vi "CheckResponse.vi"(5 "+veResponseCode":u8=160 format="%x", 7 "STP CMD":T2=130 items=["TSW_VERSION(130)"=130, "WAIT_EVENT(132)"=132, "SEQUENCER(133)"=133, "TSW_RESET(150)"=150, "CONFIG_ECU(151)"=151, "TEST_CORE (152)"=152, "TEST_WATCHDOG (153)"=153, "TEST_MONITORING (154)"=154, "READ_MEMORY (162)"=162, "WRITE_ERASE_MEMORY (164)"=164, "COMM_EXTERNAL (190)"=190, "COMM_INTERNAL (195)"=195, "GET_ANALOG_INPUT (210)"=210, "GET_DIGITAL_INPUT (211)"=211, "GET_FREQUENCY_INPUT (212)"=212, "TEST_INPUT_STRUCTURE (214)"=214, "GENERATE_OUTPUT_SIGNAL (220)"=220, "GENERATE_SYNCHRONIZED_OUTPUT_SIGNALS (221)"=221, "eDCU_Specific (250)"=250], 9 "STP Loop Data In":T1, 10 "Rx CAN frame":T4 {"payload" format="%x"; "timestamp" format="%<%.7X\n%x>T"; "type" items=["CAN Data"=0, "CAN Remote"=1, "CAN Bus Error"=2, "CAN 2.0 Data"=8, "CAN FD Data"=16, "CAN FD+BRS Data"=24, "J1939 Data"=192, "Delay"=224, "Log Trigger"=225, "Start Trigger"=226]; "identifier" format="%x"}, 11 "RxID":u32=2043 format="%x") -> (1 "STP Loop Data Out":T1, 2 "Valid Response?":bool, 3 "STP_NextState":T3=enum."Check Ack")   [LabVIEW 2023, in "HardwareAbstractionLayer_LVOOP.lvlib" / "CAN Application Protocols Lib.lvlib" / "STP Protocol.lvclass"]
uses:
  STP Protocol.lvclass
  <vilib>/xnet/xnet.llb/XNET Frame CAN.ctl
  <vilib>/xnet/xnet.llb/XNET Frame Type CAN.ctl
  Ctrls/STP States.ctl
  Ctrls/STP CMD.ctl
  Ctrls/STP Loop Data.ctl
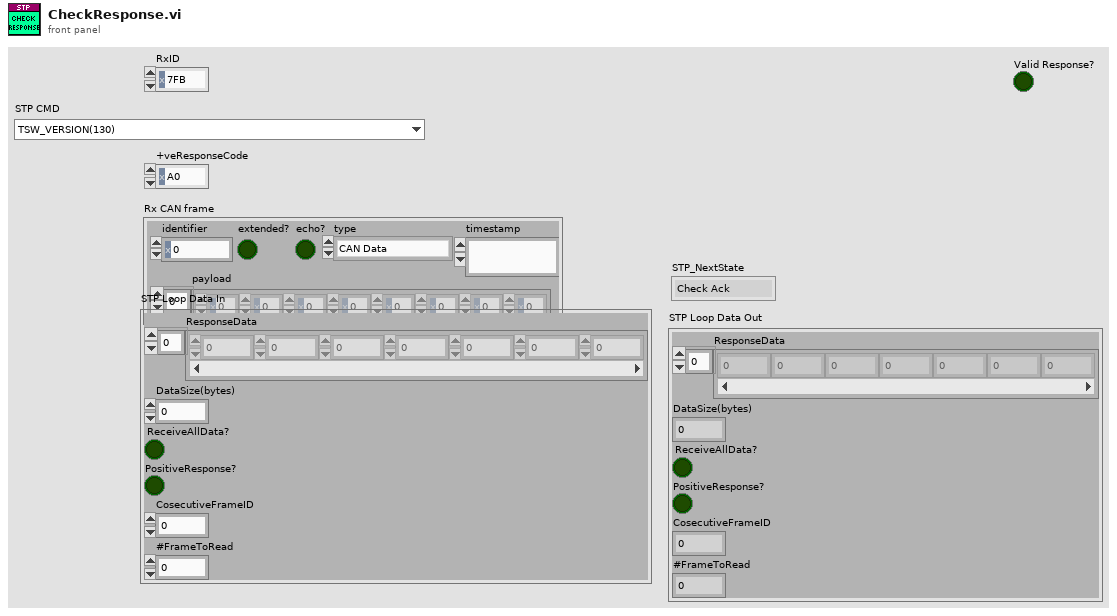
[diagram p1: front panel]
types:
  T1 = typedef "HardwareAbstractionLayer_LVOOP.lvlib/CAN Application Protocols Lib.lvlib/STP Protocol.lvclass/STP Loop Data.ctl" = cluster{"ResponseData":u8[], "DataSize(bytes)":u16, "ReceiveAllData?":bool, "PositiveResponse?":bool, "CosecutiveFrameID":fxp<+,4,4>, "#FrameToRead":i32}
  T2 = typedef "HardwareAbstractionLayer_LVOOP.lvlib/CAN Application Protocols Lib.lvlib/STP Protocol.lvclass/STP CMD.ctl" = u8
  T3 = typedef "HardwareAbstractionLayer_LVOOP.lvlib/CAN Application Protocols Lib.lvlib/STP Protocol.lvclass/STP States.ctl" = enum16{"Init", "Send Request", "Check Ack", "Send TP Frames", "Send Flow Control Frame", "Check Response", "Read TP Data", "Return Data", "Return Positive Response", "Return Error Response", "Exit"}
  T4 = typedef "XNET Frame CAN.ctl" = cluster{"timestamp":timestamp, "payload":u8[], "identifier":u32, "type":T5, "extended?":bool, "echo?":bool}
  T5 = typedef "XNET Frame Type CAN.ctl" = u8
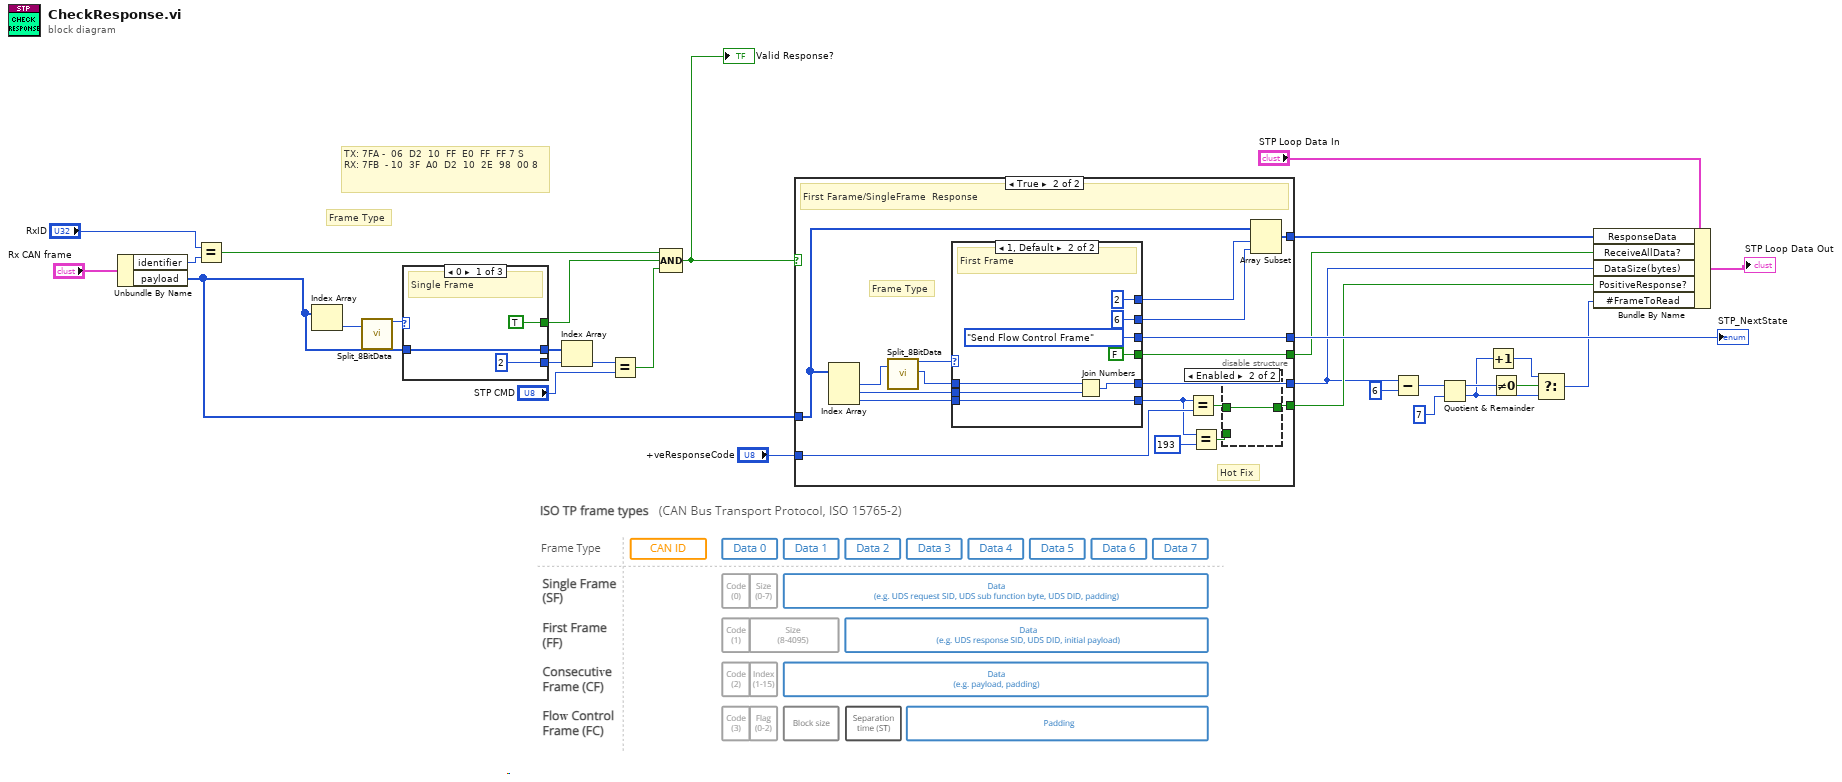
[diagram p0: block diagram]
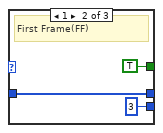
[diagram p2: hidden frame]
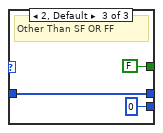
[diagram p3: hidden frame]
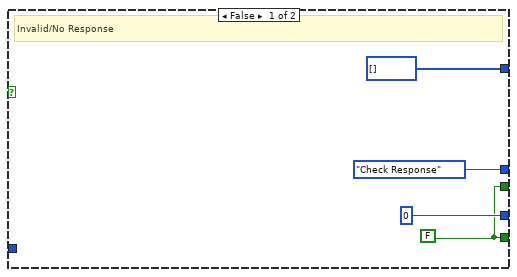
[diagram p4: hidden frame]
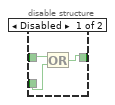
[diagram p5: hidden frame]
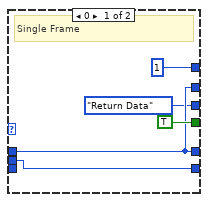
[diagram p6: hidden frame]
diagram:
  # "TX: 7FA - \t06  D2  10  FF  E0  FF  FF\t7\tS\t\nRX: 7FB\t - 10  3F  A0  D2  10  2E  98  00\t8"
  # "Frame Type"
  n1 = Unbundle By Name("Rx CAN frame") -> ("identifier"=w29:u32, "payload"=w13:u8[])
  n2 = Equal?(x="RxID", y=w29) -> (x = y?=w30:bool)
  n3 = Index Array(array=w13) -> (element=w22:u8)  [unwired: 1 in]
  n4 = call "Split_8BitData.vi"("x"=w22) -> ("hi(x)"=w21:u8)  [unwired: 17 in, 1 out]
  n5 = case shown="0" w21 {
    tunnel: [TRUE TRUE FALSE] -> w26
    tunnel: [w32 w35 w38] -> w14
    tunnel: w13 -> [w32 w35 w38]
    tunnel: [2 3 0] -> w12
    frame 0 {
      # "Single Frame"
    }
    frame 1 {
      # "First Frame(FF)"
    }
    frame 2, Default {
      # "Other Than SF OR FF"
    }
  }
  n6 = Index Array(array=w14, index=w12) -> (element=w11:u8)
  n7 = Equal?(x=w11, y="STP CMD") -> (x = y?=w10:bool)
  n8 = Compound Arithmetic op=AND(w30, w26, w10) -> (w25:bool)
  "Valid Response?" <- w25
  n9 = case shown="True" w25 {
    tunnel: [w41 w49] -> w15
    tunnel: [u8 0 ("Numeric") w58] -> w9
    tunnel: [u8[] [] ("payload") w61] -> w18
    tunnel: [w41 w60] -> w17
    tunnel: [STP_States."Check Response" w56] -> w24
    tunnel: w13 -> [_ w55]
    tunnel: "+veResponseCode" -> [_ w46]
    frame False {
      w41 = FALSE
      # "Invalid/No Response"
    }
    frame True {
      # "Hot Fix"
      # "Frame Type"
      # "First Farame/SingleFrame  Response"
      n10 = Index Array(array=w55) -> (element #1=w54:u8, element #2=w59:u8, element #3=w50:u8)  [unwired: 3 in]
      n11 = call "Split_8BitData.vi"("x"=w54) -> ("hi(x)"=w52:u8, "lo(x)"=w53:u8)  [unwired: 17 in]
      n12 = case shown="1, Default" w52 {
        tunnel: [TRUE FALSE] -> w60
        tunnel: w59 -> [w66 w77]
        tunnel: w53 -> [w69 w76]
        tunnel: [w69 w75] -> w58
        tunnel: [w69 6 ("length")] -> w57
        tunnel: [STP_States."Return Data" STP_States."Send Flow Control Frame"] -> w56
        tunnel: [1 ("index") 2 ("index")] -> w51
        tunnel: w50 -> [_ w71]
        tunnel: [w66 w71] -> w44
        frame 0 {
          # "Single Frame"
        }
        frame 1, Default {
          # "First Frame"
          n13 = Join Numbers(hi=w76, lo=w77) -> ((hi.lo)=w75:u16)
        }
      }
      n14 = Equal?(x=w44, y=w46) -> (x = y?=w48:bool)
      n15 = Equal?(x=w44, y=u8 193) -> (x = y?=w47:bool)
      n16 = disable-structure shown="Enabled" {
        disable-tunnel: [w64 w65] -> w49
        disable-tunnel: w48 -> [w63 w65]
        disable-tunnel: w47 -> [w62 _]
        frame Disabled {
          n17 = Or(x=w63, y=w62) -> (x .or. y?=w64:bool)
        }
        frame Enabled {
        }
      }
      n18 = Array Subset(array=w55, index=w51, length=w57) -> (w61:u8[])
    }
  }
  "STP_NextState" <- w24
  n19 = Subtract(x=w9, y=u16 6) -> (x-y=w7:u16)
  n20 = Quotient & Remainder(x=w7, y=u16 7) -> (x-y*floor(x/y)=w5:u16, floor(x/y)=w3:u16)
  n21 = Increment(x=w3) -> (x+1=w2:u16)
  n22 = Not Equal To 0?(x=w5) -> (x != 0?=w4:bool)
  n23 = Select(t=w2, s=w4, f=w3) -> (s? t:f=w1:u16)
  n24 = Bundle By Name(cluster="STP Loop Data In", "ResponseData"=w18, "ReceiveAllData?"=w17, "DataSize(bytes)"=w9, "PositiveResponse?"=w15, "#FrameToRead"=w1) -> (→"STP Loop Data Out":T1)
